vi "Plot Some y Cols vs x Cols.vi"(1 "Display/hide":bool[](array[boolean]), 2 "X-Axis Selection":i32=1 min=0, 3 "Input Array":dbl[][](array[numeric]) format="%.4e", 4 "Input X-Axis Array":dbl[][](array[numeric]) format="%.4e") -> (0 "Output Graph":cluster{dbl[], dbl[]}[](graph))   [LabVIEW 2025]
doc: "Plots the 2nd thru Nth columns of the matrix vs the first column in a multiplot graph. Restricted only by LV- or computer memory.\nScott Hannahs, FBNML, Jan 1992\nAuthor: Scott Hannahs <sth@magnet.fsu.edu>\n\nThis software is licensed for use under the “MIT License\"\nCopyright (c) 2025 Scott Hannahs, sth@sth@magnet.sthnet.net\n\nPermission is hereby granted, free of charge, to any person obtaining a copy of this software and associated documentation files (the \"Software\"), to deal in the Software without restriction, including without limitation the rights to use, copy, modify, merge, publish, distribute, sublicense, and/or sell copies of the Software, and to permit persons to whom the Software is furnished to do so, subject to the following conditions: The above copyright notice and this permission notice shall be included in all copies or substantial portions of the Software.\n\nTHE SOFTWARE IS PROVIDED \"AS IS\", WITHOUT WARRANTY OF ANY KIND, EXPRESS OR IMPLIED, INCLUDING BUT NOT LIMITED TO THE WARRANTIES OF MERCHANTABILITY, FITNESS FOR A PARTICULAR PURPOSE AND NONINFRINGEMENT. IN NO EVENT SHALL THE AUTHORS OR COPYRIGHT HOLDERS BE LIABLE FOR ANY CLAIM, DAMAGES OR OTHER LIABILITY, WHETHER IN AN ACTION OF CONTRACT, TORT OR OTHERWISE, ARISING FROM, OUT OF OR IN CONNECTION WITH THE SOFTWARE OR THE USE OR OTHER DEALINGS IN THE SOFTWARE."
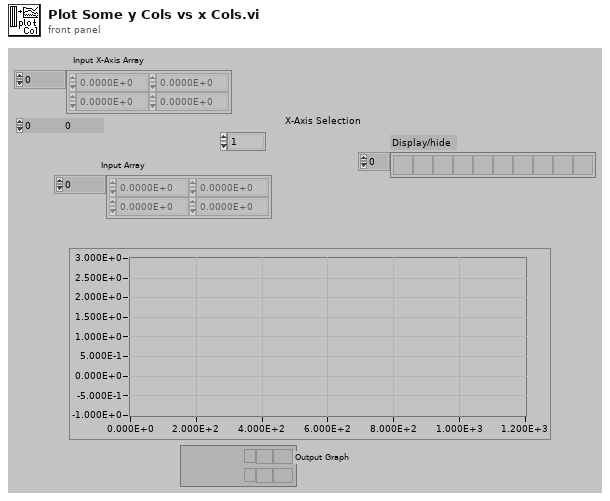
[diagram p1: front panel]
types:
  T1 = cluster{"Input X-Axis Array":dbl[], "Input Array":dbl[]}
  T2 = cluster{"Input X-Axis Array":dbl[], "Input Array":dbl[]}[]
  T3 = cluster{"Index Array":dbl[], "Input Array":dbl[]}
  T4 = cluster{"Index Array":dbl[], "Input Array":dbl[]}[]
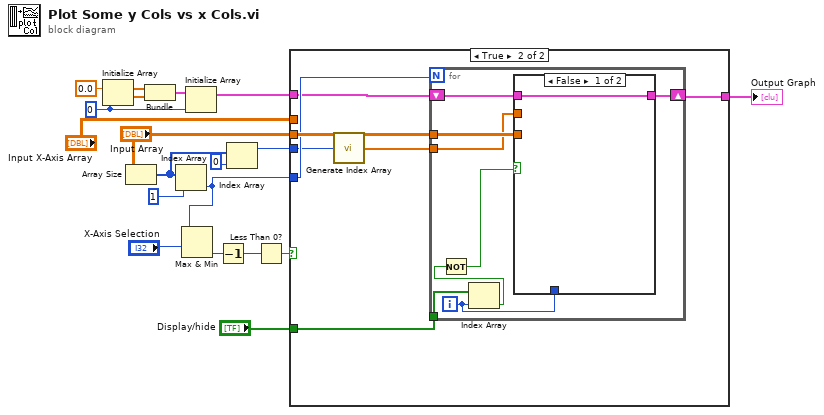
[diagram p0: block diagram]
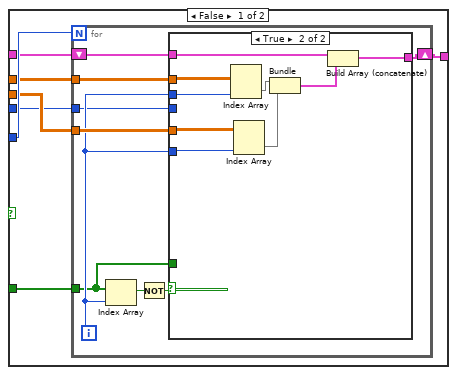
[diagram p2: hidden frame]
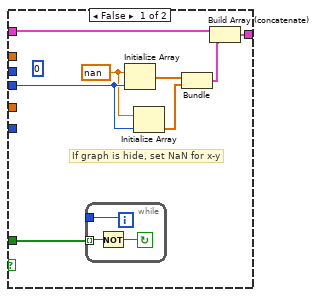
[diagram p3: hidden frame]
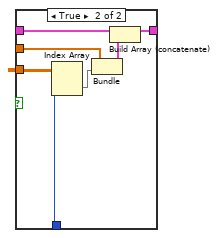
[diagram p4: hidden frame]
diagram:
  w7 = 0
  n1 = Initialize Array(0.0, w7) -> (w10:dbl[])
  n2 = Array Size(array="Input Array") -> (size(s)=w5:i32[])
  n3 = Bundle(w10, w10) -> (w9:cluster{dbl[], dbl[]})  [unwired: 1 in]
  n4 = Index Array(array=w5, index=1) -> (element=w12:i32)
  n5 = Max & Min(x=w12, y="X-Axis Selection") -> (min(x,y)=w16:i32)  [unwired: 1 out]
  n6 = Initialize Array(w9, w7) -> (w8:cluster{dbl[], dbl[]}[])
  n7 = Decrement(x=w16) -> (x-1=w1:i32)
  n8 = Index Array(array=w5, index=0) -> (element=w4:i32)
  n9 = Less Than 0?(x=w1) -> (x < 0?=w17:bool)
  n10 = case shown="True" w17 {
    tunnel: w12 -> [w23 w59]
    tunnel: "Display/hide" -> [w24 w60]
    tunnel: [w25 w58] -> w3
    tunnel: "Input Array" -> [w21 w61]
    tunnel: w8 -> [w22 w57]
    tunnel: w4 -> [w19 w56]
    tunnel: "Input X-Axis Array" -> [w20 _]
    frame False {
      n11 = for {
        N: w23 -> [_]
        shift-right: [w33] -> w25
        shift-left: w22 -> [w34]
        tunnel: w24 -> [w27]
        tunnel: w21 -> [w31]
        tunnel: w20 -> [w30]
        tunnel: w19 -> [w26]
        i -> [w29]
        n12 = Index Array(array=w27, index=w29) -> (element=w32:bool)
        n13 = Not(x=w32) -> (.not. x?=w28:bool)
        n14 = case shown="True" w28 {
          tunnel: [w40 w53] -> w33
          tunnel: w34 -> [w41 w54]
          tunnel: w31 -> [_ w49]
          tunnel: w29 -> [_ w48]
          tunnel: w29 -> [_ w47]
          tunnel: w30 -> [_ w46]
          tunnel: w27 -> [w42 _]
          tunnel: w26 -> [w38 _]
          frame False {
            w35 = nan ("element")
            (unwired) 0
            # "If graph is hide, set NaN for x-y"
            n15 = while {
              tunnel: [w43] -> _
              tunnel: w42 -> [w44] mode=indexing
              i -> [w43]
              stop <- w45 continue-if-true
              n16 = Not(x=w44) -> (.not. x?=w45:bool)
            }
            n17 = Initialize Array(w35, w38) -> (w39:dbl[])
            n18 = Initialize Array(w35, w38) -> (w37:dbl[])
            n19 = Bundle(w39, w37) -> (w36:cluster{dbl[], dbl[]})  [unwired: 1 in]
            n20 = Build Array (concatenate)(w41, w36) -> (w40:cluster{dbl[], dbl[]}[])
          }
          frame True {
            n21 = Index Array(array=w46, index (col)=w47) -> (element=w51:dbl[])  [unwired: 1 in]
            n22 = Index Array(array=w49, index (col)=w48) -> (element=w50:dbl[])  [unwired: 1 in]
            n23 = Bundle("Input X-Axis Array"=w51, "Input Array"=w50) -> (w52:T1)  [unwired: 1 in]
            n24 = Build Array (concatenate)(w54, w52) -> (w53:T2)
          }
        }
      }
    }
    frame True {
      n25 = call "Generate Index Array.vi"("Size"=w56) -> ("Index Array"=w55:dbl[])
      n26 = for {
        N: w59 -> [_]
        shift-right: [w68] -> w58
        shift-left: w57 -> [w67]
        tunnel: w60 -> [w66]
        tunnel: w61 -> [w69]
        tunnel: w55 -> [w63]
        i -> [w62]
        n27 = Index Array(array=w66, index=w62) -> (element=w65:bool)
        n28 = Not(x=w65) -> (.not. x?=w64:bool)
        n29 = case shown="False" w64 {
          tunnel: w62 -> [_ w74]
          tunnel: w69 -> [_ w75]
          tunnel: [w70 w76] -> w68
          tunnel: w67 -> [w70 w77]
          tunnel: w63 -> [_ w71]
          frame False {
          }
          frame True {
            n30 = Index Array(array=w75, index (col)=w74) -> (element=w73:dbl[])  [unwired: 1 in]
            n31 = Bundle("Index Array"=w71, "Input Array"=w73) -> (w72:T3)  [unwired: 1 in]
            n32 = Build Array (concatenate)(w77, w72) -> (w76:T4)
          }
        }
      }
    }
  }
  "Output Graph" <- w3
